vi "Read Map of Messages to Value Indexes.vi"(8 "error in":errorcluster, 11 "Rx execution unit in":refnum<class "Rx Execution Unit.lvclass">) -> (0 "error out":errorcluster, 2 "map of messages to value indexes":T1, 3 "Rx execution unit out":refnum<class "Rx Execution Unit.lvclass">)   [LabVIEW 2020, in "AIM MIL-STD-1553 Engine.lvlib" / "Implementation.lvlib" / "Rx Execution Unit.lvclass"]
uses:
  Rx Execution Unit.lvclass
  Shared/Address.ctl
  Shared/Terminal Endpoint.ctl
  Shared/Parameter Definition.ctl
  Shared/Message Type.ctl
  Shared/Message Definition.ctl
  Message Map Value.ctl
  Shared/Message Map Key.ctl
  Shared/Map of Messages to Value Indexes.ctl
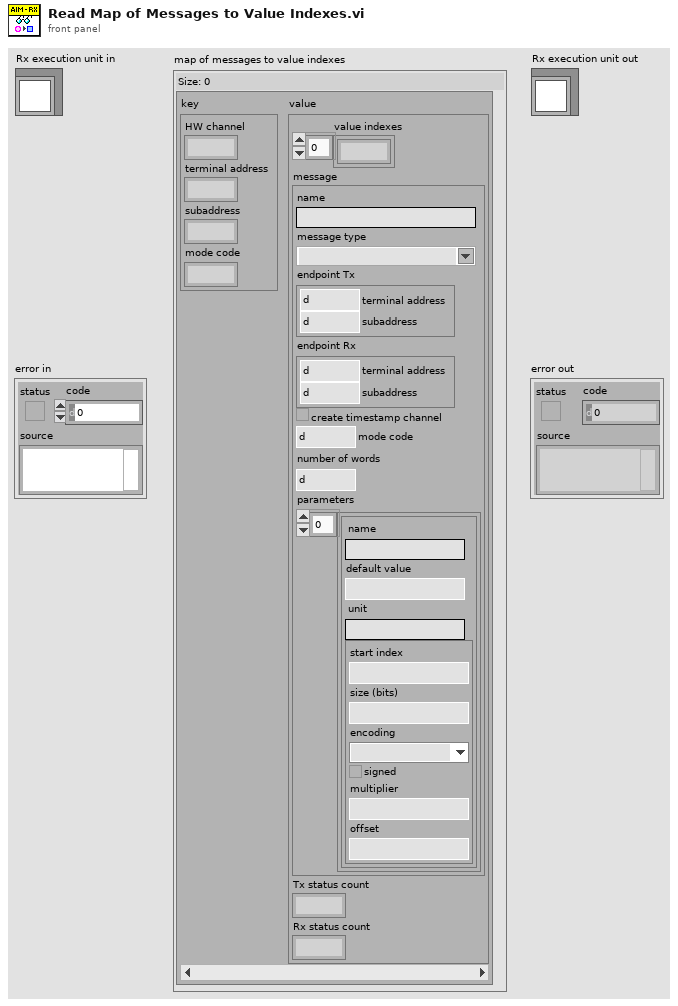
[diagram p1: front panel]
types:
  T1 = typedef "Map of Messages to Value Indexes.ctl" = map{T2, T3}
  T2 = typedef "Message Map Key.ctl" = cluster{"HW channel":u16, "terminal address":u16, "subaddress":u16, "mode code":u16}
  T3 = typedef "AIM MIL-STD-1553 Engine.lvlib/Implementation.lvlib/Rx Execution Unit.lvclass/Message Map Value.ctl" = cluster{"value indexes":i32[], "message":T4, "Tx status count":i32, "Rx status count":i32}
  T4 = typedef "Message Definition.ctl" = cluster{"name":string, "message type":T5, "endpoint Tx":T6, "endpoint Rx":T6, "create timestamp channel":bool, "mode code":u16, "number of words":u16, "parameters":cluster{"name":string, "default value":dbl, "unit":string, "parameter definition":T8}[]}
  T5 = typedef "Message Type.ctl" = string
  T6 = typedef "Terminal Endpoint.ctl" = cluster{"terminal address":T7, "subaddress":T7}
  T7 = typedef "Address.ctl" = u16
  T8 = typedef "Parameter Definition.ctl" = cluster{"start index":i32, "size (bits)":i32, "encoding":enum16{"BNR", "BCD", "Discrete"}, "signed":bool, "multiplier":dbl, "offset":dbl}
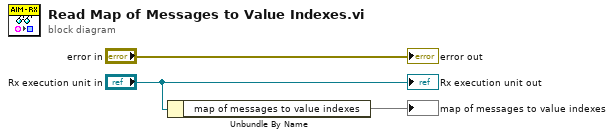
[diagram p0: block diagram]
diagram:
  n1 = Unbundle By Name("Rx execution unit in") -> ("map of messages to value indexes"=→"map of messages to value indexes":T1)
  "error out" <- "error in"
  "Rx execution unit out" <- "Rx execution unit in"
